vi "Close.vi"(8 "error in (no error)":errorcluster, 11 "ManageControls in":refnum<class "Controls_Mgr.lvclass">) -> (0 "error out":errorcluster, 3 "ManageControls out":refnum<class "Controls_Mgr.lvclass">)   [LabVIEW 2015, in "Generic Module Library.lvlib" / "Template G_Module.lvlib" / "Controls_Mgr.lvclass"]
uses:
  Controls_Mgr.lvclass
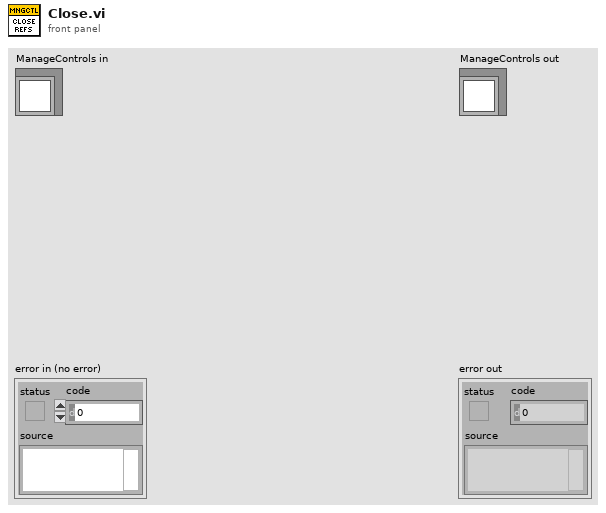
[diagram p1: front panel]
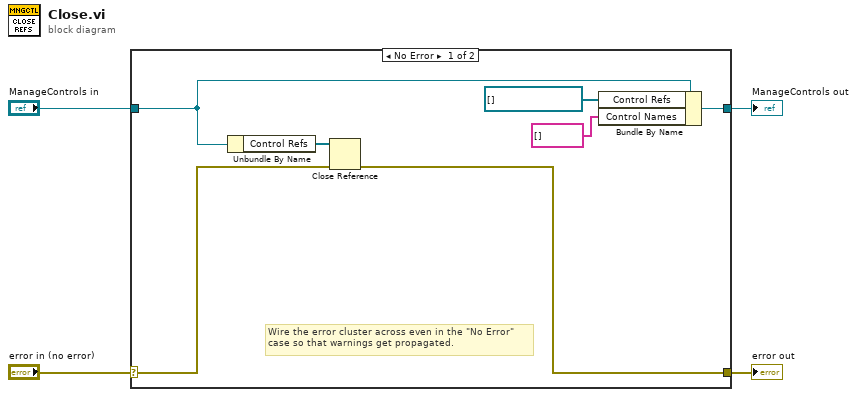
[diagram p0: block diagram]
diagram:
  n1 = case shown="No Error" "error in (no error)" {
    selector: "error in (no error)" -> [w10 w13]
    tunnel: [w9 w13] -> w3
    tunnel: [w8 w12] -> w1
    tunnel: "ManageControls in" -> [w7 w12]
    frame No Error {
      # "Wire the error cluster across even in the \"No Error\"\ncase so that warnings get propagated."
      n2 = Unbundle By Name(w7) -> ("Control Refs"=w11:refnum<vi>[])
      n3 = Close Reference(reference=w11, error in (no error)=w10) -> (error out=w9:errorcluster)
      n4 = Bundle By Name(cluster=w7, "Control Refs"=refnum<vi>[] [], "Control Names"=string[] []) -> (w8:refnum<class "Controls_Mgr.lvclass">)
    }
    frame Error {
    }
  }
  "error out" <- w3
  "ManageControls out" <- w1
